vi "Select Reference Dialog.vi"() -> (2 "Reference Type":enum16{"VI", "Class"}(ring))   [LabVIEW 2016]
panel:
  in  "Boolean":bool
  in  "Enum":enum16{"VI", "Class"}(ring)
  # "Select Reference Type"
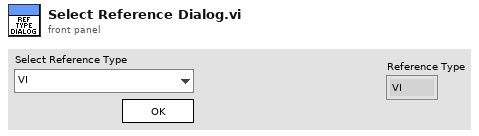
[diagram p1: front panel]
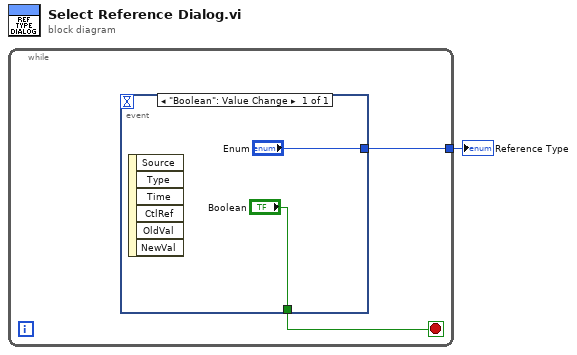
[diagram p0: block diagram]
diagram:
  n1 = while {
    tunnel: [w2] -> w1
    stop <- w3 stop-if-true
    n2 = event shown="[0] \"Boolean\": Value Change" {
      selector: _ -> [_]
      dyn-events: _ -> [_]
      timeout: _ -> [_]
      tunnel: ["Boolean"] -> w3
      tunnel: ["Enum"] -> w2
      event "Boolean": Value Change {
        n3 = event-data() -> ()  [unwired: 1 in, 6 out]
      }
    }
  }
  "Reference Type" <- w1
